vi "Msg Loop.vi"(11 "Actor in":refnum<class "Actor.lvclass">) -> ()   [LabVIEW 2021, in "AAM.lvlib" / "Actor.lvclass"]
uses:
  Actor.lvclass
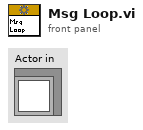
[diagram p1: front panel]
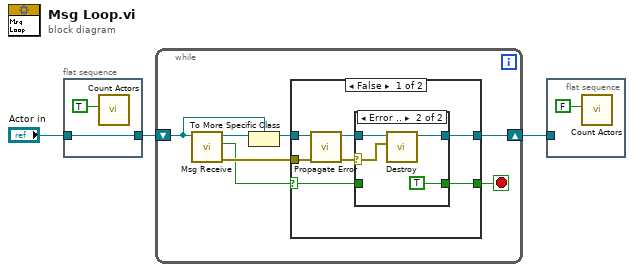
[diagram p0: block diagram]
diagram:
  n1 = flat-sequence {
    tunnel: "Actor in" -> [w5]
    tunnel: [w5] -> w3
    frame #0 {
      n2 = call "Count Actors.vi"("Increment?"=TRUE) -> ()  [unwired: 11 in]
    }
  }
  n3 = while {
    shift-right: [w12] -> w2
    shift-left: w3 -> [w7]
    stop <- w11 stop-if-true
    n4 = call-dynamic "Msg Receive.vi"("Msg Receive in"=w7) -> ("error out"=w9:errorcluster, "Destroy Self?"=w6:bool, "Msg Receive out"=w10:refnum<class "Msg Receive.lvclass">)  [unwired: 8 in]
    n5 = To More Specific Class(target class=w7, reference=w10) -> (specific class reference=w8:refnum<class "Actor.lvclass">)  [unwired: 1 in, 1 out]
    n6 = case shown="False" w6 {
      selector: w6 -> [w17 w26]
      tunnel: w9 -> [w15 _]
      tunnel: [w19 w27] -> w12
      tunnel: w8 -> [w16 w27]
      tunnel: [w18 w26] -> w11
      frame False {
        n7 = call-dynamic "Propagate Error.vi"("error in (no error)"=w15, "Propagate Error in"=w16) -> ("error out"=w13:errorcluster, "Propagate Error out"=w14:refnum<class "Actor.lvclass">)  [unwired: 8 in]
        n8 = case shown="Error .." w13 {
          selector: w13 -> [_ w22]
          tunnel: [w21 w23] -> w19
          tunnel: w14 -> [w21 w24]
          tunnel: [w20 TRUE] -> w18
          tunnel: w17 -> [w20 _]
          frame No Error {
          }
          frame Error {
            n9 = call-dynamic "Destroy.vi"("Error"=w22, "Destroy in"=w24) -> ("Destroy out"=w23:refnum<class "Actor.lvclass">)  [unwired: 8 in, 1 out]
          }
        }
      }
      frame True {
      }
    }
  }
  n10 = flat-sequence {
    tunnel: w2 -> [_]
    frame #0 {
      n11 = call "Count Actors.vi"("Increment?"=FALSE) -> ()  [unwired: 11 in]
    }
  }
